vi "OpenWindowAndSendData(SubVI).vi"(8 "Error In":errorcluster, 10 "Combo Box":refnum<vi>, 11 "Cluster in":refnum<vi>) -> (0 "Error Out":errorcluster)   [LabVIEW 2018]
uses:
  Windows/Settings/GraphSettings/GraphSettings_STM.ctl
  Windows/Settings/GraphSettings/GraphSettings_ITEM.ctl
  CTL/STM GRAPH.ctl
  CTL/Graph settings.ctl
  CTL/Line.ctl
  Windows/Settings/View.ctl
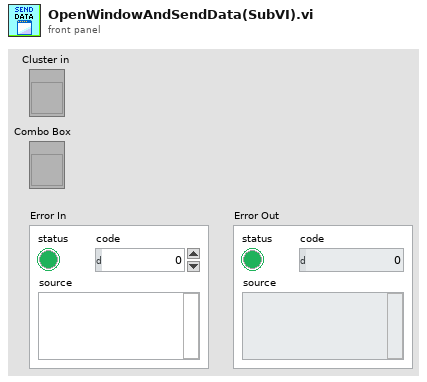
[diagram p1: front panel]
types:
  T1 = typedef "GraphSettings_STM.ctl" = cluster{"main stm":T2, "STM Graph":T3}
  T2 = typedef "GraphSettings_ITEM.ctl" = enum16{"idle", "init", "close", "_____ SETTINGS _____ ", "Receive Data", "Send Data", "Change Line", "Delete Line", "Add Line", "Find Max", "Change Color", "Choice Line"}
  T3 = typedef "STM GRAPH.ctl" = cluster{"Graph settings":T4, "Lines":T5[], "Data":string}
  T4 = typedef "Graph settings.ctl" = cluster{"Axis X Min":dbl, "Axis X Name":string, "Axis X Max":dbl, "Axis Y Min":dbl, " Axis Y Name":string, "Axis Y Max":dbl, "Autoscale":enum16{"Yes", "No", "Only Oy", "Only Ox"}, "Choice Line":dbl}
  T5 = typedef "Line.ctl" = cluster{"Width":dbl, "Color":i64, "Array Oy":dbl[], "Array Ox":dbl[], "Name":string, "Plot Visible":T6}
  T6 = typedef "View.ctl" = bool
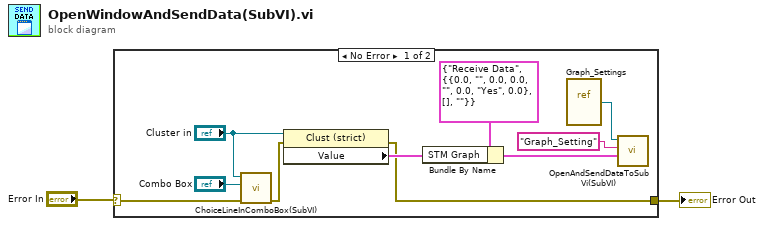
[diagram p0: block diagram]
diagram:
  n1 = case shown="No Error" "Error In" {
    selector: "Error In" -> [w6 w13]
    tunnel: [w5 w13] -> w1
    frame No Error {
      n2 = call "ChoiceLineInComboBox(SubVI).vi"("Error In"=w6, "ComboBox in"="Combo Box", "Cluster in"="Cluster in") -> ("Error Out"=w12:errorcluster)  [unwired: 8 in]
      n3 = property on="Property Node" class="Clust (strict)"(reference="Cluster in", error in=w12) -> (error out=w5:errorcluster, "Value"=w8:T3)  [unwired: 1 out]
      n4 = Bundle By Name(cluster=T1 {"main stm"=enum."Receive Data", "STM Graph"={"Graph settings"={"Axis X Min"=0.0, "Axis X Name"="", "Axis X Max"=0.0, "Axis Y Min"=0.0, " Axis Y Name"="", "Axis Y Max"=0.0, "Autoscale"=enum."Yes", "Choice Line"=0.0}, "Lines"=[], "Data"=""}} ("MOKO_SE_STM"), "STM Graph"=w8) -> (w9:T1)
      n5 = vi-ref "Graph_Settings.vi"() -> (w10:refnum<vi>)
      n6 = call "OpenAndSendDataToSubVi(SubVI).vi"("reference"=w10, "Control Name"="Graph_Setting", "element"=w9) -> ()  [unwired: 8 in]
    }
    frame Error {
    }
  }
  "Error Out" <- w1
